vi "Move_Arm_to_Card.vi"(9 "index":i32=19, 10 "error in":errorcluster, 11 "Machine In":refnum<visa-resource-name>) -> (2 "error out":errorcluster, 3 "Machine Out":refnum<visa-resource-name>)   [LabVIEW 2018]
doc: "Example interface for controlling uArm Swift Pro."
panel:
  in  "Write Buffer":string="G90 G0 X1\n"
  out "read buffer":string
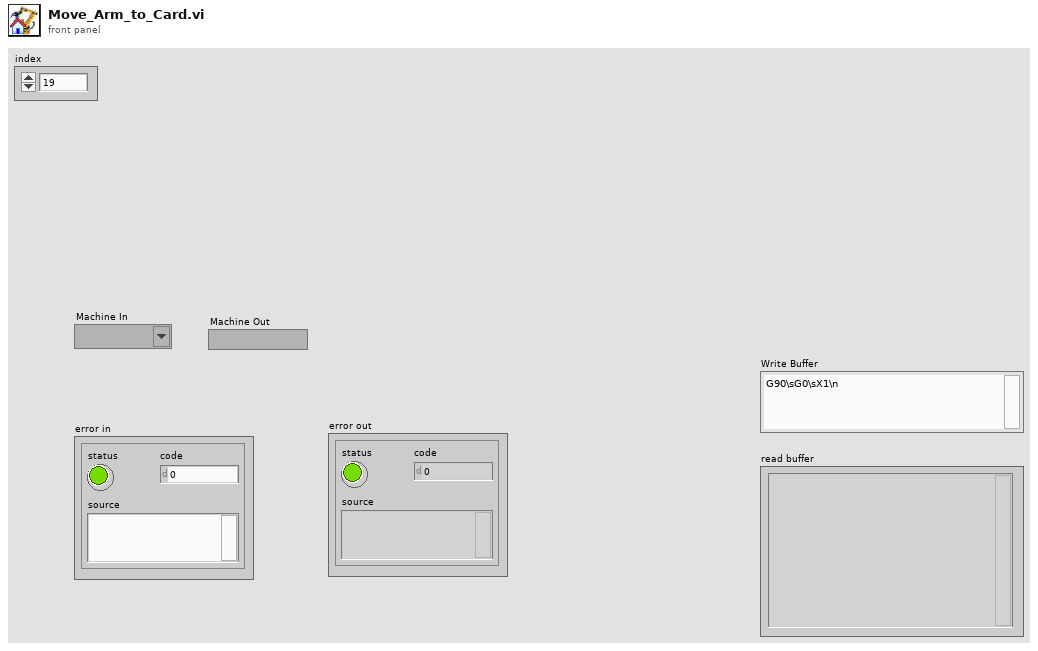
[diagram p1: front panel]
types:
  T1 = cluster{"Numeric Control":dbl, "Numeric Control":dbl}[]
  T2 = cluster{"Numeric Control":dbl, "Numeric Control":dbl}
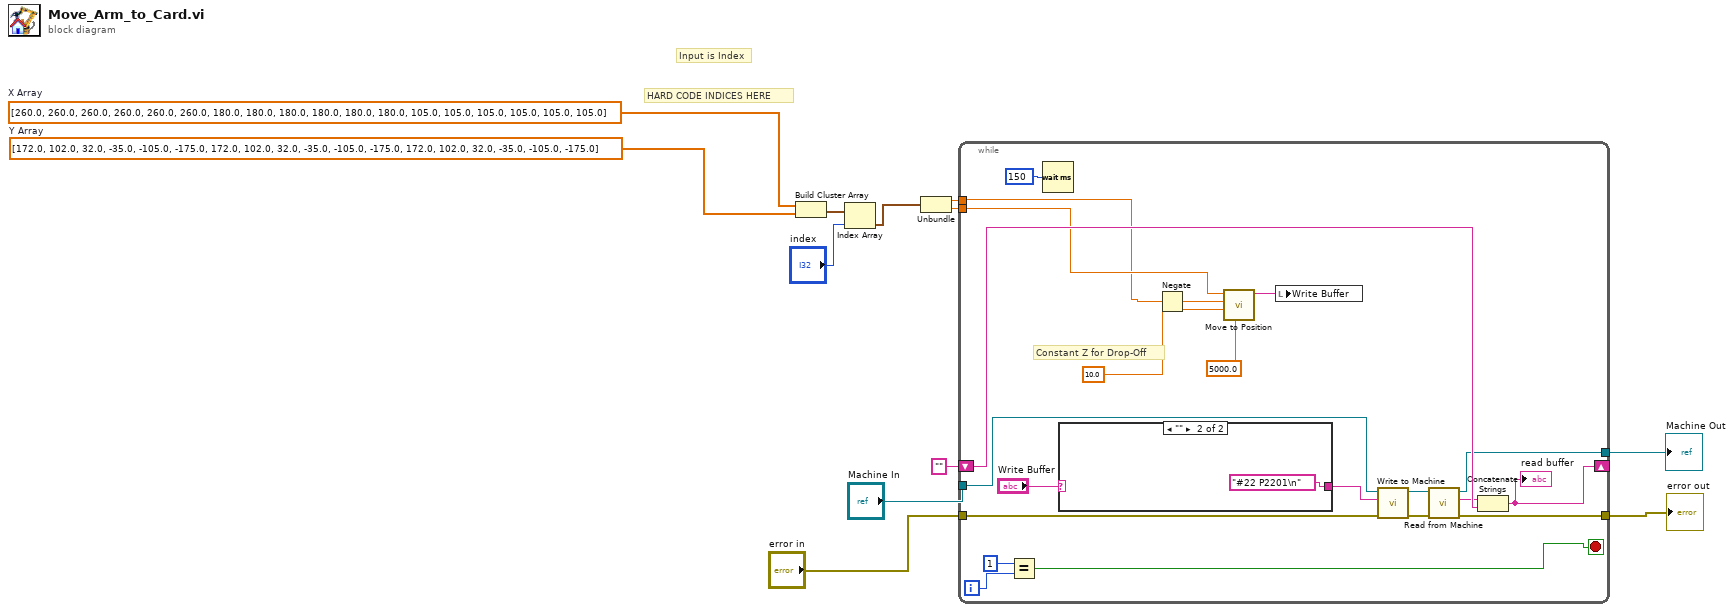
[diagram p0: block diagram]
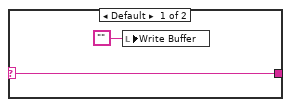
[diagram p2: hidden frame]
diagram:
  w10 = dbl[] [172.0, 102.0, 32.0, -35.0, -105.0, -175.0, 172.0, 102.0, 32.0, -35.0, -105.0, -175.0, 172.0, 102.0, 32.0, -35.0, -105.0, -175.0]  # Y Array
  w11 = dbl[] [260.0, 260.0, 260.0, 260.0, 260.0, 260.0, 180.0, 180.0, 180.0, 180.0, 180.0, 180.0, 105.0, 105.0, 105.0, 105.0, 105.0, 105.0]  # X Array
  # "HARD CODE INDICES HERE"
  # "Input is Index"
  n1 = Build Cluster Array(w11, w10) -> (w9:T1)
  n2 = Index Array(array=w9, index="index") -> (element=w8:T2)
  n3 = Unbundle(w8) -> ("Numeric Control"=w6:dbl, "Numeric Control"=w7:dbl)
  n4 = while {
    tunnel: "Machine In" -> [w30]
    tunnel: "error in" -> [w27]
    shift-right: [w28] -> _
    shift-left: "" -> [w29]
    tunnel: [w26] -> w2
    tunnel: [w22] -> w1
    tunnel: w7 -> [w18]
    tunnel: w6 -> [w17]
    i -> [w15]
    stop <- w13 stop-if-true
    # "Constant Z for Drop-Off"
    n5 = Equal?(x=1, y=w15) -> (x = y?=w13:bool)
    n6 = Wait (ms)(milliseconds to wait=u32 150) -> ()  [unwired: 1 out]
    n7 = case shown="\"\"" "Write Buffer" {
      selector: "Write Buffer" -> [w35 _]
      tunnel: [w35 "#22 P2201\n"] -> w32
      frame Default {
        n8 = local write "Write Buffer"("") -> ()
      }
      frame "" {
      }
    }
    n9 = Negate(x=w17) -> (-x=w20:dbl)
    n10 = call "Move to Position.vi"("Speed"=5000.0, "Z-Position"=10.0, "Y-Position"=w20, "X-Position"=w18) -> ("G-Code String"=w21:string)  [unwired: 7 in]
    n11 = local write "Write Buffer"(w21) -> ()
    n12 = call "Write to Machine .vi"("error in (no error)"=w27, "G-Code String In"=w32, "Machine In"=w30) -> ("error out"=w24:errorcluster, "Machine Out"=w23:refnum<visa-resource-name>)  [unwired: 7 in]
    n13 = call "Read from Machine.vi"("error in (no error)"=w24, "Machine In"=w23) -> ("error out"=w22:errorcluster, "read buffer"=w25:string, "Machine Out"=w26:refnum<visa-resource-name>)  [unwired: 7 in]
    n14 = Concatenate Strings(w25, w29) -> (w28:string)
    "read buffer" <- w28
  }
  "Machine Out" <- w2
  "error out" <- w1
